vi "Forward To File Writer.vi"(8 "error in (no error)":errorcluster, 9 "Await Completion?":bool, 10 "Actor in":refnum<class "Actor.lvclass">, 11 "Response Msg in":refnum<class "Response Msg.lvclass">) -> (0 "error out":errorcluster, 2 "Actor out":refnum<class "Actor.lvclass">)   [LabVIEW 2020, in "File Writer.lvlib"]
doc: "Send the Response Msg to all File Writers. If Await Completion is TRUE the message will await a reply. Any recieved data will not be published."
uses:
  File Writer.lvlib
  PPL/HDH.Actor Framework.Core.Publisher.lvlibp/Messages/Response Msg/Response Msg.lvclass
  PPL/HDH.Actor Framework.Core.Actor.lvlibp/1abvi3w/vi.lib/ActorFramework/Actor/Actor.lvclass
  PPL/HDH.Actor Framework.Core.Publisher.lvlibp/Messages/Response Msg/Response Core/Controls/Ctl_SendFunction.ctl
  File Writer/File Writer.lvclass
  PPL/HDH.Actor Framework.Core.Publisher.lvlibp/Publisher Messages/Targetted Msg/Targetted Msg.lvclass
  C:/Current projects/WS/PPL/HDH.Actor Framework.Core.Publisher.lvlibp/Publisher Messages/Sender Msg/Sender Msg.lvclass
  PPL/HDH.Actor Framework.Core.Publisher.lvlibp
  C:/Current projects/WS/PPL/HDH.Actor Framework.Core.Actor.lvlibp/1abvi3w/vi.lib/ActorFramework/Actor/Actor.lvclass
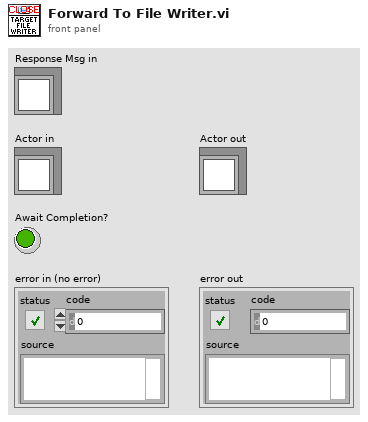
[diagram p1: front panel]
types:
  T1 = typedef "HDH.Actor Framework.Core.Publisher.lvlibp/Ctl_SendFunction.ctl" = enum16{"Send and Forget", "Request Reply", "Await Reply"}
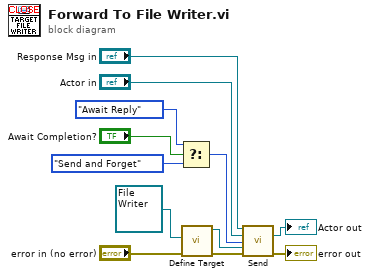
[diagram p0: block diagram]
diagram:
  n1 = Select(t=Ctl_SendFunction."Await Reply" ("Send Function"), s="Await Completion?", f=Ctl_SendFunction."Send and Forget" ("Send Function")) -> (s? t:f=w6:T1)
  n2 = call "Define Target.vi"("error in (no error)"="error in (no error)", "Target Actor"=refnum<class "File Writer.lvclass"> refnum ("File Writer.lvlib:File Writer.lvclass")) -> ("error out"=w7:errorcluster, "Targetted Msg out"=w3:refnum<class "Targetted Msg.lvclass">)  [unwired: 8 in]
  n3 = call "Send.vi"("Response Msg in"="Response Msg in", "Actor in"="Actor in", "Send Function"=w6, "Sender (publish)"=w3, "error in (no error)"=w7) -> ("Actor out"=→"Actor out":refnum<class "Actor.lvclass">, "error out"=→"error out":errorcluster)  [unwired: 6 in, 3 out]
